vi "-8002 PCAN_ERROR_OVERRUN CAN Controller was read too late--error.vi"(8 "error in":errorcluster, 11 "Channel":string) -> (0 "error out":errorcluster, 2 "Error Code":i32)   [LabVIEW 2018, in "PCANBasic.lvlib"]
uses:
  PCANBasic.lvlib
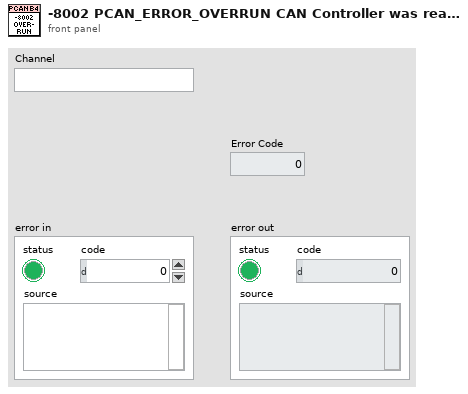
[diagram p1: front panel]
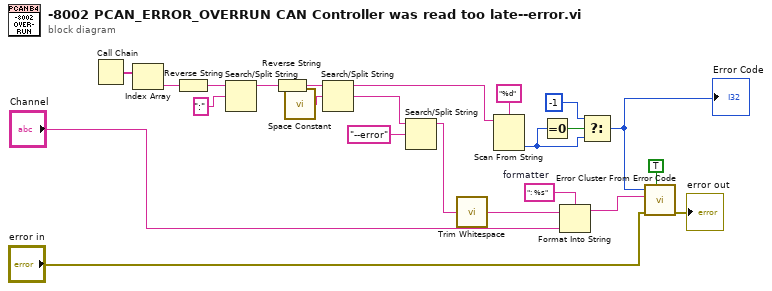
[diagram p0: block diagram]
diagram:
  w20 = ": %s"  # formatter
  n1 = Call Chain() -> (call chain=w13:string[])
  n2 = Index Array(array=w13) -> (element=w7:string)  [unwired: 1 in]
  n3 = Reverse String(1:w7) -> (0:w12:string)
  n4 = Search/Split String(string=w12, search string/char (-)=":") -> (substring before match=w11:string)  [unwired: 1 in, 2 out]
  n5 = Reverse String(1:w11) -> (0:w9:string)
  n6 = call <vilib>:"Space Constant.vi"() -> ("String"=w8:string)
  n7 = Search/Split String(string=w9, search string/char (-)=w8) -> (substring before match=w6:string, match + rest of string=w4:string)  [unwired: 1 in, 1 out]
  n8 = Search/Split String(string=w4, search string/char (-)="--error") -> (substring before match=w3:string)  [unwired: 1 in, 2 out]
  n9 = call <vilib>:"Trim Whitespace.vi"("string"=w3) -> ("trimmed string"=w2:string)  [unwired: 1 in]
  n10 = Scan From String(format string="%d", input string=w6) -> (output 1=w16:i32)  [unwired: 3 in, 3 out]
  n11 = Equal To 0?(x=w16) -> (x = 0?=w17:bool)
  n12 = Format Into String(format string=w20, initial string=w2, "Channel") -> (resulting string=w21:string)  [unwired: 1 in, 1 out]
  n13 = Select(t=-1, s=w17, f=w16) -> (s? t:f=w14:i32)
  "Error Code" <- w14
  n14 = call <vilib>:"Error Cluster From Error Code.vi"("show call chain? (False)"=TRUE, "error in (no error)"="error in", "error message (\"\")"=w21, "error code (0)"=w14) -> ("error out"=→"error out":errorcluster)  [unwired: 5 in]
